vi "IntersecaoAreaQuadrada.vi"(7 "Pos entrada":dbl[](array[numeric]) format="%#_13g", 11 "geometry":T1) -> (3 "Pos de interseção":dbl[](array[numeric]) format="%#_13g")   [LabVIEW 2017]
uses:
  Core/Field Size.ctl
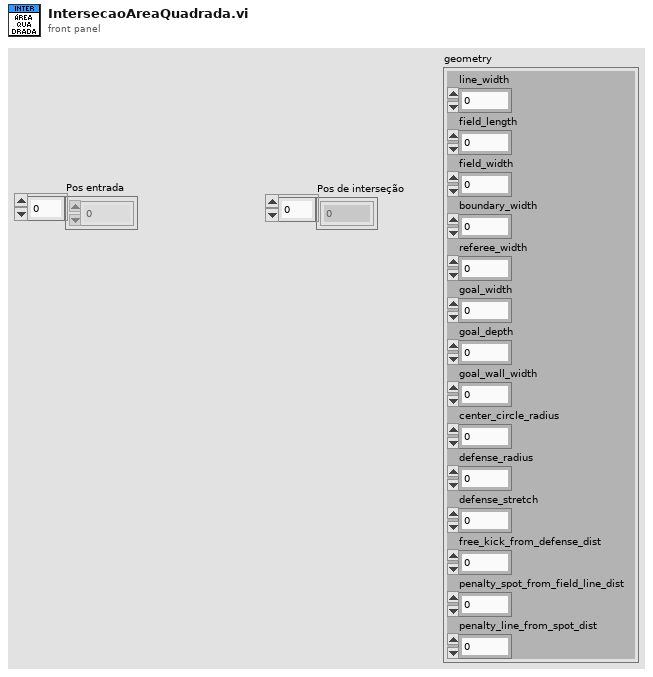
[diagram p1: front panel]
types:
  T1 = typedef "Field Size.ctl" = cluster{"line_width":u32, "field_length":u32, "field_width":u32, "boundary_width":u32, "referee_width":u32, "goal_width":u32, "goal_depth":u32, "goal_wall_width":u32, "center_circle_radius":u32, "defense_radius":u32, "defense_stretch":u32, "free_kick_from_defense_dist":u32, "penalty_spot_from_field_line_dist":u32, "penalty_line_from_spot_dist":u32}
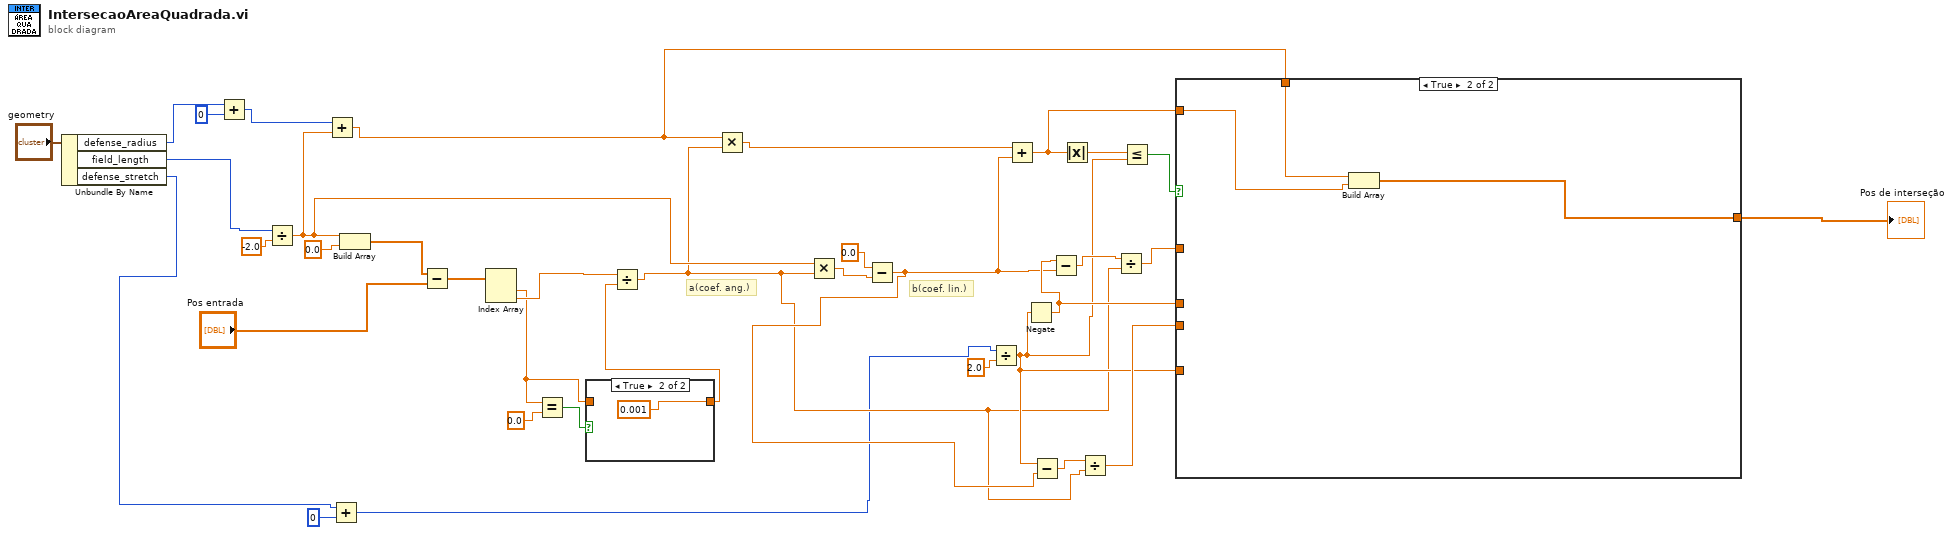
[diagram p0: block diagram]
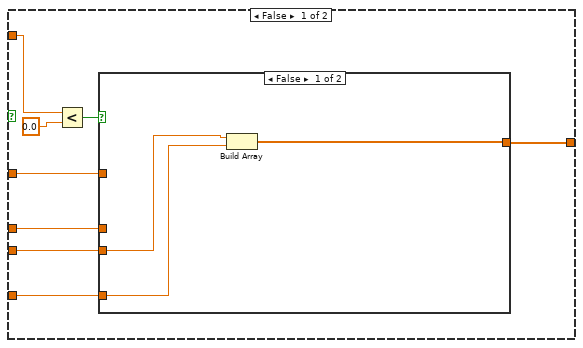
[diagram p3: hidden frame]
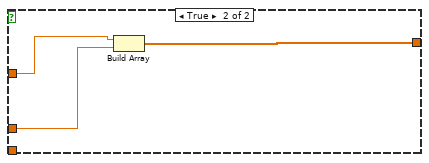
[diagram p4: hidden frame]
diagram:
  # "b(coef. lin.)"
  # "a(coef. ang.)"
  n1 = Unbundle By Name("geometry") -> ("defense_radius"=w6:u32, "field_length"=w7:u32, "defense_stretch"=w3:u32)
  n2 = Add(x=w6, y=u32 0) -> (x+y=w5:u32)
  n3 = Divide(x=w7, y=-2.0) -> (x/y=w28:dbl)
  n4 = Add(x=w5, y=w28) -> (x+y=w22:dbl)
  n5 = Add(x=w3, y=u32 0) -> (x+y=w1:u32)
  n6 = Build Array(w28, 0.0 ("element")) -> (w33:dbl[])
  n7 = Subtract(x=w33, y="Pos entrada") -> (x-y=w32:dbl[])
  n8 = Index Array(array=w32) -> (element #1=w10:dbl, element #2=w31:dbl)  [unwired: 2 in]
  n9 = Equal?(x=w10, y=0.0) -> (x = y?=w11:bool)
  n10 = case shown="True" w11 {
    tunnel: w10 -> [w37 _]
    tunnel: [w37 0.001] -> w9
    frame False {
    }
    frame True {
    }
  }
  n11 = Divide(x=w31, y=w9) -> (x/y=w13:dbl)
  n12 = Multiply(x=w22, y=w13) -> (x*y=w27:dbl)
  n13 = Multiply(x=w28, y=w13) -> (x*y=w30:dbl)
  n14 = Subtract(x=0.0, y=w30) -> (x-y=w17:dbl)
  n15 = Divide(x=w1, y=2.0) -> (x/y=w14:dbl)
  n16 = Add(x=w27, y=w17) -> (x+y=w23:dbl)
  n17 = Negate(x=w14) -> (-x=w18:dbl)
  n18 = Subtract(x=w14, y=w17) -> (x-y=w16:dbl)
  n19 = Subtract(x=w18, y=w17) -> (x-y=w20:dbl)
  n20 = Absolute Value(x=w23) -> (abs(x)=w26:dbl)
  n21 = Divide(x=w16, y=w13) -> (x/y=w15:dbl)
  n22 = Divide(x=w20, y=w13) -> (x/y=w19:dbl)
  n23 = Less Or Equal?(x=w26, y=w14) -> (x <= y?=w24:bool)
  n24 = case shown="True" w24 {
    tunnel: w23 -> [w46 w55]
    tunnel: w22 -> [_ w54]
    tunnel: [w41 w53] -> w21
    tunnel: w19 -> [w43 _]
    tunnel: w18 -> [w42 _]
    tunnel: w15 -> [w40 _]
    tunnel: w14 -> [w39 _]
    frame False {
      n25 = Less?(x=w46, y=0.0) -> (x < y?=w44:bool)
      n26 = case shown="False" w44 {
        tunnel: w43 -> [_ w52]
        tunnel: w42 -> [_ w51]
        tunnel: [w47 w50] -> w41
        tunnel: w40 -> [w49 _]
        tunnel: w39 -> [w48 _]
        frame False {
          n27 = Build Array(w49, w48) -> (w47:dbl[])
        }
        frame True {
          n28 = Build Array(w52, w51) -> (w50:dbl[])
        }
      }
    }
    frame True {
      n29 = Build Array(w54, w55) -> (w53:dbl[])
    }
  }
  "Pos de interseção" <- w21
